vi "set_pixel_frequency.vi"(8 "error in (no error)":errorcluster, 10 "pixel frequency":dbl[unit], 11 "FPGAWrapperDL090211Galvo_grabber in":refnum<class "FPGAWrapperMM140723Galvo.lvclass">) -> (0 "error out":errorcluster, 3 "FPGAWrapperDL090211Galvo_grabber out":refnum<class "FPGAWrapperMM140723Galvo.lvclass">)   [LabVIEW 2010, in "FPGAWrapperMM140723Galvo.lvclass"]
uses:
  FPGAWrapperMM140723Galvo.lvclass
  FPGAWrapperMM140723Galvo.lvclass/FPGAWrapperMM140723Galvo.ctl
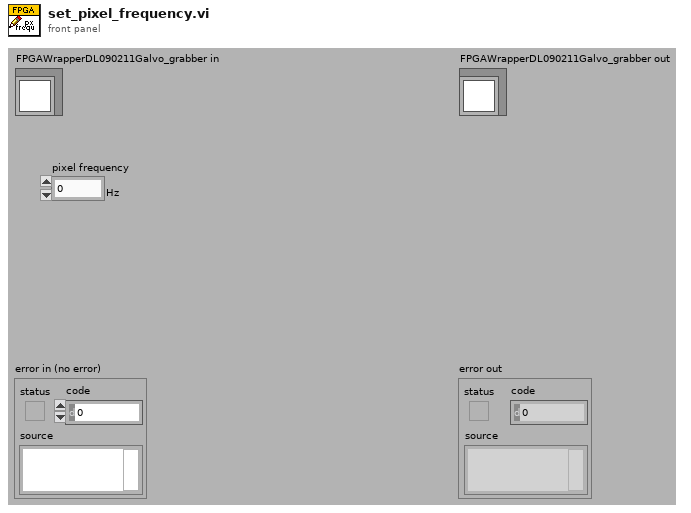
[diagram p1: front panel]
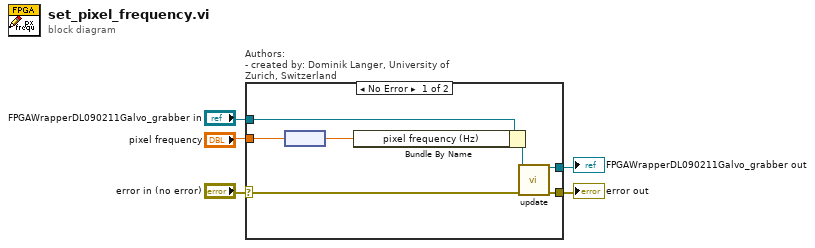
[diagram p0: block diagram]
diagram:
  n1 = case "Authors: \n- created by: Dominik Langer, University of Zurich, Switzerland" shown="No Error" "error in (no error)" {
    selector: "error in (no error)" -> [w8 w14]
    tunnel: [w9 w13] -> w1
    tunnel: [w7 w14] -> w2
    tunnel: "FPGAWrapperDL090211Galvo_grabber in" -> [w12 w13]
    tunnel: "pixel frequency" -> [w11 _]
    frame No Error {
      n2 = node(w11) -> (w6:dbl)
      n3 = Bundle By Name(cluster=w12, "pixel frequency (Hz)"=w6) -> (w10:refnum<class "FPGAWrapperMM140723Galvo.lvclass">)
      n4 = call-dynamic "update.vi"("error in (no error)"=w8, "FPGAWrapperDL120115Galvo in"=w10) -> ("error out"=w7:errorcluster, "FPGAWrapperDL120115Galvo out"=w9:refnum<class "FPGAWrapperMM140723Galvo.lvclass">)  [unwired: 8 in]
    }
    frame Error {
    }
  }
  "error out" <- w2
  "FPGAWrapperDL090211Galvo_grabber out" <- w1
